vi "Get Image Timings.vi"(8 "error in (no error)":errorcluster, 10 "Kinetic Series Lenght":u16, 11 "Header in":refnum<class "Header.lvclass">) -> (0 "error out":errorcluster, 3 "Header out":refnum<class "Header.lvclass">)   [LabVIEW 2018, in "Header.lvclass"]
uses:
  Header.lvclass
  Header.lvclass/Header.ctl
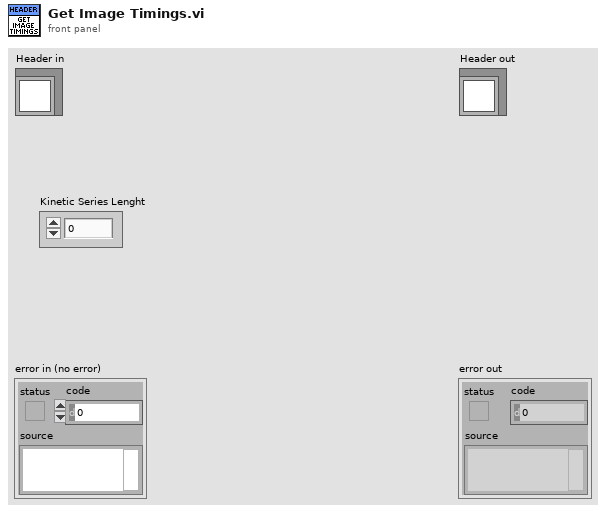
[diagram p1: front panel]
types:
  T1 = typedef "SYSTEMTIME structure typedef.ctl" = cluster{"Year":u16, "Month":u16, "DayOfWeek":u16, "Date":u16, "Hour":u16, "Minute":u16, "Second":u16, "Milliseconds":u16}
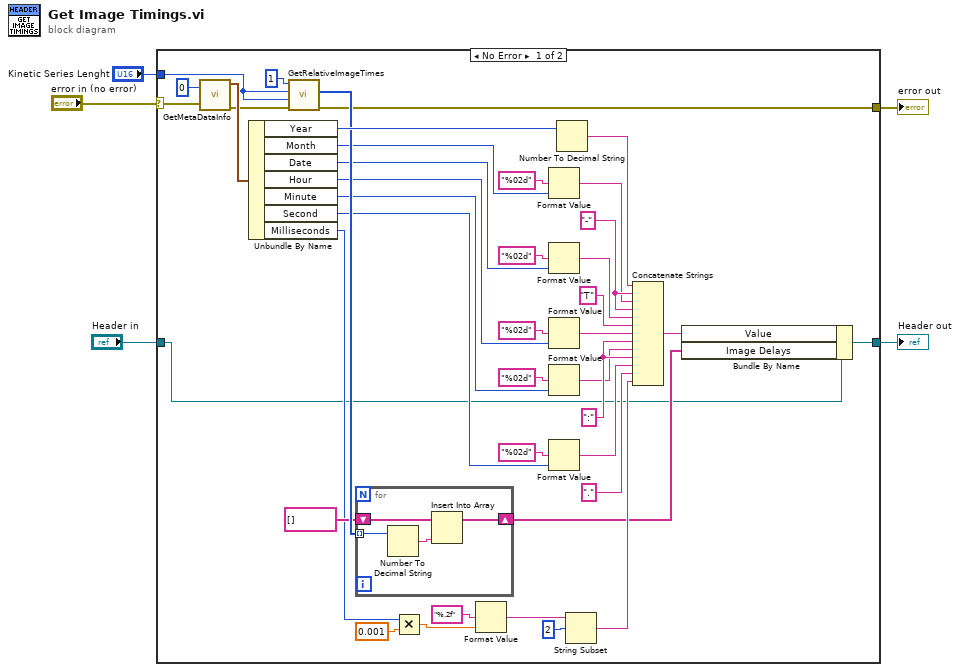
[diagram p0: block diagram]
diagram:
  n1 = case shown="No Error" "error in (no error)" {
    selector: "error in (no error)" -> [w12 w52]
    tunnel: [w11 w52] -> w3
    tunnel: [w10 w51] -> w2
    tunnel: "Header in" -> [w7 w51]
    tunnel: "Kinetic Series Lenght" -> [w8 _]
    frame No Error {
      w38 = ":"
      w40 = "-"
      n2 = call <userlib>:"GetMetaDataInfo.vi"("index"=0, "error in (no error)"=w12) -> ("SYSTEMTIME"=w46:T1, "error out"=w43:errorcluster)  [unwired: 2 out]
      n3 = Unbundle By Name(w46) -> ("Year"=w44:u16, "Month"=w24:u16, "Date"=w23:u16, "Hour"=w22:u16, "Minute"=w21:u16, "Second"=w20:u16, "Milliseconds"=w14:u16)
      n4 = call <userlib>:"GetRelativeImageTimes.vi"("error in (no error)"=w43, "size"=w8, "last"=w8, "first"=u32 1) -> ("error out"=w11:errorcluster, "arr"=w42:u64[])  [unwired: 5 in, 1 out]
      n5 = for {
        shift-right: [w47] -> w9
        shift-left: string[] [] -> [w48]
        tunnel: w42 -> [w50] mode=indexing
        n6 = Number To Decimal String(number=w50) -> (decimal integer string=w49:string)  [unwired: 1 in]
        n7 = Insert Into Array(array=w48, new element=w49) -> (w47:string[])  [unwired: 1 in]
      }
      n8 = Multiply(x=w14, y=0.001) -> (x*y=w19:dbl)
      n9 = Format Value(format string="%.2f", value (0)=w19) -> (output string=w18:string)  [unwired: 1 in]
      n10 = Format Value(format string="%02d", value (0)=w24) -> (output string=w33:string)  [unwired: 1 in]
      n11 = Format Value(format string="%02d", value (0)=w23) -> (output string=w31:string)  [unwired: 1 in]
      n12 = Format Value(format string="%02d", value (0)=w22) -> (output string=w29:string)  [unwired: 1 in]
      n13 = Format Value(format string="%02d", value (0)=w21) -> (output string=w27:string)  [unwired: 1 in]
      n14 = Format Value(format string="%02d", value (0)=w20) -> (output string=w25:string)  [unwired: 1 in]
      n15 = Number To Decimal String(number=w44) -> (decimal integer string=w45:string)  [unwired: 1 in]
      n16 = String Subset(string=w18, offset (0)=2) -> (substring=w13:string)  [unwired: 1 in]
      n17 = Concatenate Strings(w45, w40, w33, w40, w31, "T", w29, w38, w27, w38, w25, ".", w13) -> (w6:string)
      n18 = Bundle By Name(cluster=w7, "Value"=w6, "Image Delays"=w9) -> (w10:refnum<class "Header.lvclass">)
    }
    frame Error {
    }
  }
  "error out" <- w3
  "Header out" <- w2
